vi "Save Seq.vi"(8 "error in":errorcluster, 11 "Sequence in":refnum<class "Sequence.lvclass">) -> (0 "error out":errorcluster, 3 "Sequence out":refnum<class "Sequence.lvclass">)   [LabVIEW 2019]
uses:
  Sequence.lvclass
  C:/Program Files (x86)/National Instruments/LabVIEW 2019/vi.lib/ActorFramework/Actor/Actor.lvclass
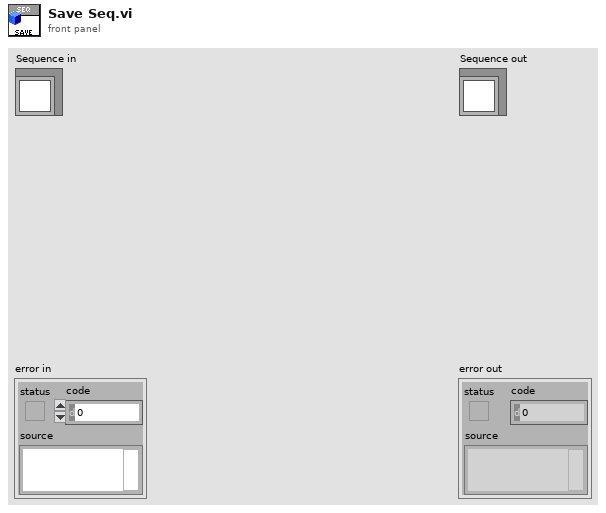
[diagram p1: front panel]
types:
  T1 = enum16{"Left Button", "Center Button", "Right Button", "Window Close"}
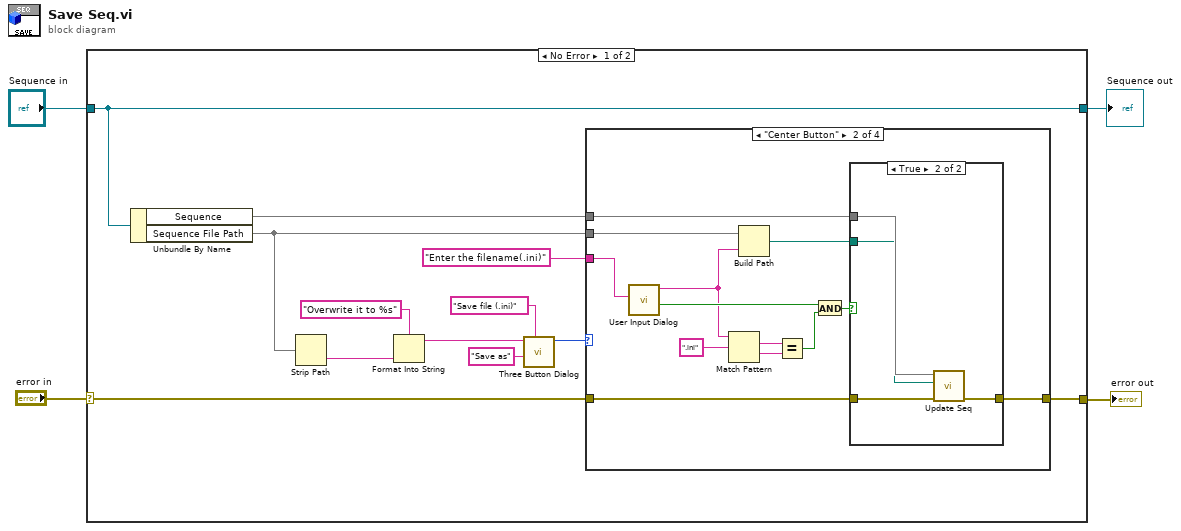
[diagram p0: block diagram]
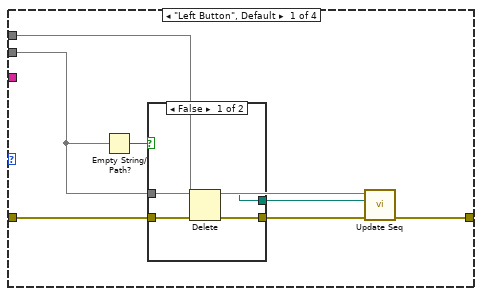
[diagram p2: hidden frame]
diagram:
  n1 = case shown="No Error" "error in" {
    selector: "error in" -> [w7 w50]
    tunnel: [w8 w50] -> w3
    tunnel: [w6 w49] -> w1
    tunnel: "Sequence in" -> [w6 w49]
    frame No Error {
      n2 = Unbundle By Name(w6) -> ("Sequence"=w5, "Sequence File Path"=w15)
      n3 = Strip Path(path=w15) -> (name=w16:string)  [unwired: 1 out]
      n4 = Format Into String(format string="Overwrite it to %s", w16) -> (resulting string=w9:string)  [unwired: 2 in, 1 out]
      n5 = call <vilib>:"Three Button Dialog.vi"("Window Title (\"\")"="Save file (.ini)" ("Window Title (\"\")"), "Center Button Text (\"No\")"="Save as" ("Center Button Text (\"No\")"), "message"=w9) -> ("Which Button?"=w13:T1)  [unwired: 8 in]
      n6 = case shown="\"Center Button\"" w13 {
        tunnel: "Enter the filename(.ini)" ("Message title") -> [_ w41 _ _]
        tunnel: w15 -> [w21 w33 _ _]
        tunnel: w7 -> [w22 w35 w47 w48]
        tunnel: [w18 w31 w47 w48] -> w8
        tunnel: w5 -> [w20 w30 _ _]
        frame "Left Button", Default {
          n7 = Empty String/Path?(string/path=w21) -> (empty?=w23:bool)
          n8 = case shown="False" w23 {
            tunnel: w21 -> [w27 w28]
            tunnel: w22 -> [w26 w29]
            tunnel: [w25 w28] -> w17
            tunnel: [w24 w29] -> w19
            frame False {
              n9 = Delete(path (use dialog)=w27, error in=w26) -> (deleted path=w25:path, error out=w24:errorcluster)  [unwired: 3 in, 1 out]
            }
            frame True {
            }
          }
          n10 = call "Update Seq.vi"("Error In"=w19, "file path"=w17, "Sequence in"=w20) -> ("error out"=w18:errorcluster)  [unwired: 7 in, 1 out]
        }
        frame "Center Button" {
          w38 = ".ini" ("regular expression")
          n11 = call "User Input Dialog.vi"("Message title"=w41) -> ("OK?"=w37:bool, "Message out"=w34:string)  [unwired: 7 in, 1 out]
          n12 = Match Pattern(string=w34, regular expression=w38) -> (match substring=w40:string)  [unwired: 1 in, 3 out]
          n13 = Build Path(base path=w33, name or relative path=w34) -> (appended path=w32:path)
          n14 = Equal?(x=w40, y=w38) -> (x = y?=w39:bool)
          n15 = And(x=w37, y=w39) -> (x .and. y?=w36:bool)
          n16 = case shown="True" w36 {
            tunnel: w32 -> [_ w43]
            tunnel: w35 -> [w42 w46]
            tunnel: [w42 w45] -> w31
            tunnel: w30 -> [_ w44]
            frame False {
            }
            frame True {
              n17 = call "Update Seq.vi"("Error In"=w46, "file path"=w43, "Sequence in"=w44) -> ("error out"=w45:errorcluster)  [unwired: 7 in, 1 out]
            }
          }
        }
        frame "Right Button" {
        }
        frame "Window Close" {
        }
      }
    }
    frame Error {
    }
  }
  "error out" <- w3
  "Sequence out" <- w1
